vi "Split byte.vi"(0 "x":u8 format="%08b") -> (1 "hi(x)":fxp<+,4,4> format="%04b", 2 "lo(x)":fxp<+,4,4> format="%04b")   [LabVIEW 2013]
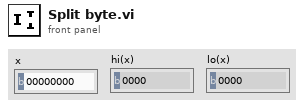
[diagram p1: front panel]
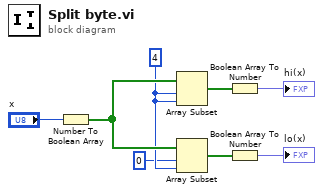
[diagram p0: block diagram]
diagram:
  w2 = 4 ("length")
  n1 = Number To Boolean Array(number="x") -> (Boolean array=w6:bool[])
  n2 = Array Subset(array=w6, index=w2, length=w2) -> (w7:bool[])
  n3 = Array Subset(array=w6, index=0, length=w2) -> (w4:bool[])
  n4 = Boolean Array To Number(Boolean array=w7) -> (number=→"hi(x)":fxp<+,4,4>)
  n5 = Boolean Array To Number(Boolean array=w4) -> (number=→"lo(x)":fxp<+,4,4>)
